vi "Query_Windows_Volume.vi"(8 "error in (no error)":errorcluster, 10 "nFolder":u8, 11 "Dest_NI_MSIPath in":refnum<class "Dest_NI_MSIPath.lvclass">) -> (0 "error out":errorcluster, 3 "Dest_NI_MSIPath out":refnum<class "Dest_NI_MSIPath.lvclass">)   [LabVIEW 2020, in "Dest_NI_MSIPath.lvclass"]
uses:
  <vilib>/AppBuilder/IB_Classes/Dest_NI_MSIPath/Dest_NI_MSIPath.lvclass
  <vilib>/AppBuilder/IB_Classes/Dest_NI_MSIPath/Dest_NI_MSIPath.lvclass/Dest_NI_MSIPath.ctl
  <vilib>/AppBuilder/IB_Classes/Destination/niLabel/niLabel.lvclass
  e:/builds/penguin/labview/branches/2020/dev/dist/vi.lib/AppBuilder/IB_Classes/Destination/niLabel/niLabel.lvclass
  e:/builds/penguin/labview/branches/2020/dev/dist/vi.lib/AppBuilder/IB_Classes/Destination/IB_Destination.lvclass
  e:/builds/penguin/labview/branches/2020/dev/dist/vi.lib/AppBuilder/IB_Classes/Dest_NI_MSIPath/Dest_NI_MSIPath.lvclass
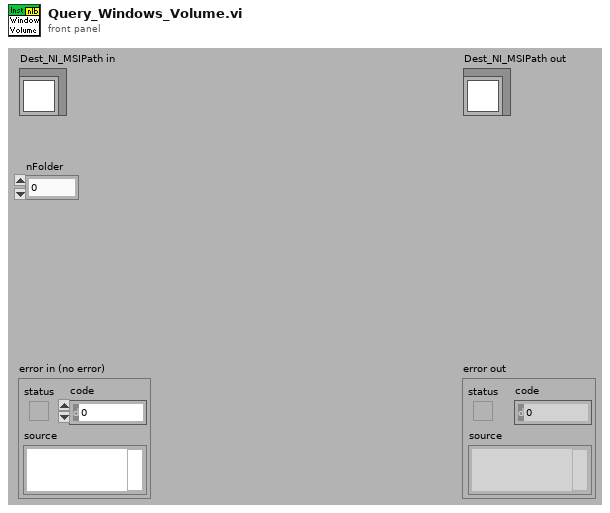
[diagram p1: front panel]
types:
  T1 = typedef "IB_Dest_niLabel.ctl" = cluster{"local path":path}
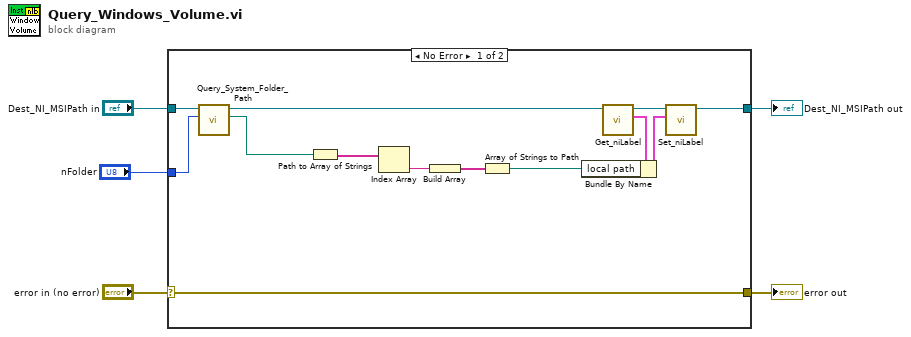
[diagram p0: block diagram]
diagram:
  n1 = case shown="No Error" "error in (no error)" {
    selector: "error in (no error)" -> [w18 w20]
    tunnel: [w18 w20] -> w4
    tunnel: [w7 w19] -> w2
    tunnel: "Dest_NI_MSIPath in" -> [w17 w19]
    tunnel: "nFolder" -> [w16 _]
    frame No Error {
      n2 = call <vilib>:"Query_System_Folder_Path.vi"("nFolder"=w16, "Dest_NI_MSIPath in"=w17) -> ("path"=w12:path, "Dest_NI_MSIPath out"=w9:refnum<class "Dest_NI_MSIPath.lvclass">)  [unwired: 7 in, 1 out]
      n3 = Path to Array of Strings(0:w12) -> (2:w15:string[])  [unwired: 1 out]
      n4 = Index Array(array=w15) -> (element=w14:string)  [unwired: 1 in]
      n5 = Build Array(w14) -> (w13:string[])
      n6 = Array of Strings to Path(0:w13) -> (2:w6:path)  [unwired: 1 in]
      n7 = call <vilib>:"Get_niLabel.vi"("niLabel in"=w9) -> ("data"=w11:T1, "niLabel out"=w8:refnum<class "Dest_NI_MSIPath.lvclass">)  [unwired: 8 in, 1 out]
      n8 = Bundle By Name(cluster=w11, "local path"=w6) -> (w10:T1)
      n9 = call <vilib>:"Set_niLabel.vi"("data"=w10, "niLabel in"=w8) -> ("niLabel out"=w7:refnum<class "Dest_NI_MSIPath.lvclass">)  [unwired: 8 in, 1 out]
    }
    frame Error {
    }
  }
  "error out" <- w4
  "Dest_NI_MSIPath out" <- w2
